vi "FUG_MagnetPS.Contents.vi"   [LabVIEW 2014, in "FUG_MagnetPS.lvlib"]
uses:
  FUG_MagnetPS.lvlib
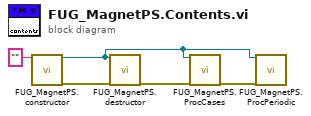
[diagram p0: block diagram]
diagram:
  n1 = call "FUG_MagnetPS.constructor.vi"("name"="") -> ("i ref out"=w3:refnum<vi>, "error out"=w5:errorcluster)  [unwired: 16 in, 1 out]
  n2 = call "FUG_MagnetPS.destructor.vi"("i ref in"=w3, "error in (no error)"=w5) -> ("error out"=w2:errorcluster)  [unwired: 17 in]
  n3 = call "FUG_MagnetPS.ProcCases.vi"("i ref in"=w3, "error in (no error)"=w2) -> ("error out"=w1:errorcluster)  [unwired: 15 in, 2 out]
  n4 = call "FUG_MagnetPS.ProcPeriodic.vi"("i ref in"=w3, "error in (no error)"=w1) -> ()  [unwired: 15 in, 3 out]
